vi "timeDvsfreqD_demo.vi"() -> ()   [LabVIEW 2009]
uses:
  <vilib>/imath/engines/lvmath2/RunTimeEngine/ErrorHandling/NIMS_Finalize Error.vi
  <vilib>/imath/engines/lvmath2/RunTimeEngine/Parser/MC_Version.vi
  <vilib>/imath/engines/lvmath2/RunTimeEngine/NodeEndStatement/NIMS_NodeEndStatement_Output.vi
  <instcachedir>/0/NIMS_NodeEndStatement_Output_53EC0D466D134D7ABD903AC30B43404B.lvgen/NIMS_NodeEndStatement_Output_53EC0D466D134D7ABD903AC30B43404B_001.vi
  <vilib>/imath/engines/lvmath/Functions/Error Handling/MergeErrorsWrapper.vi
  <vilib>/imath/engines/lvmath2/RunTimeEngine/NodeEndStatement/NIMS_NodeEndStatement_Get Vector.vi
  <instcachedir>/0/NIMS_NodeEndStatement_Get Vector_708AE642CFEE4B9892E482CBBBA3A4D6.lvgen/NIMS_NodeEndStatement_Get Vector_708AE642CFEE4B9892E482CBBBA3A4D6_000.vi
  <instcachedir>/0/NIMS_NodeEndStatement_Get Vector_708AE642CFEE4B9892E482CBBBA3A4D6.lvgen/NIMS_NodeEndStatement_Get Vector_708AE642CFEE4B9892E482CBBBA3A4D6_001.vi
  <vilib>/imath/engines/lvmath2/RunTimeEngine/RangeToken/NIMS_Range.vi
  <instcachedir>/0/NIMS_Range_08574DECC23E450FAF0AC0BC39E6BEA7.lvgen/NIMS_Range_08574DECC23E450FAF0AC0BC39E6BEA7_001.vi
  <vilib>/imath/engines/lvmath/Plug In/_Char/NIMS_CH_character datatype.ctl
  <vilib>/imathl/engines/lvmath/Functions/Error Handling/Create Error.vi
  <vilib>/imath/engines/lvmath2/RunTimeEngine/BuiltInFunctions/random/NIMS_random.vi
  <vilib>/imath/engines/lvmath/Plug In/_Char/NIMS_CH_Character RV to String.vi
  <vilib>/imath/engines/lvmath/Functions/Error Handling/MC_Error Cluster From Error Code.vi
  <vilib>/imath/engines/lvmath2/RunTimeEngine/BuiltInFunctions/abs/NIMS_abs(signed).vi
  <instcachedir>/0/NIMS_abs(signed)_C4FCB8E6058B49B797C7C8D53CA5F6EC.lvgen/NIMS_abs(signed)_C4FCB8E6058B49B797C7C8D53CA5F6EC_000.vi
  <vilib>/imath/engines/lvmath2/RunTimeEngine/BuiltInFunctions/fft/NIMS_fft(GV).vi
  <instcachedir>/0/NIMS_fft(GV)_4C6467FC22F84E4BA42517A07EF978B0.lvgen/NIMS_fft(GV)_4C6467FC22F84E4BA42517A07EF978B0_001.vi
  <vilib>/imath/engines/lvmath2/RunTimeEngine/ArithmeticOperatorToken/NIMS_ArithmeticOperator_plus.vi
  <instcachedir>/0/NIMS_ArithmeticOperator_plus_48B9519178ED42D7840F01273E784BFE.lvgen/NIMS_ArithmeticOperator_plus_48B9519178ED42D7840F01273E784BFE_008.vi
  <instcachedir>/0/NIMS_abs(signed)_C4FCB8E6058B49B797C7C8D53CA5F6EC.lvgen/NIMS_abs(signed)_C4FCB8E6058B49B797C7C8D53CA5F6EC_002.vi
  <vilib>/imath/engines/lvmath2/RunTimeEngine/BuiltInFunctions/fft/NIMS_fft(GM).vi
  <instcachedir>/0/NIMS_fft(GM)_D61006EB97DF48D4B7BC0A22887DF931.lvgen/NIMS_fft(GM)_D61006EB97DF48D4B7BC0A22887DF931_000.vi
panel:
  in  "nmag":dbl=1e-06 caption="Order of \nMagnitude \nof the \nNoise" format="%#_6p"
  in  "M1":dbl=10.0
  in  "N1":dbl=256.0
  out "Both Signals (Frequency Domain)":cluster{dbl[], dbl[]}[](graph)
  out "Both Signals (Time Domain)":cluster{dbl[], dbl[]}[](graph)
  out "Total Signal (Frequency Domain)":dbl[](graph)
  out "Total Signal (Time Domain)":dbl[](graph)
  out "Desired Signal (Frequency Domain)":dbl[](graph)
  out "Desired Signal (Time Domain)":dbl[](graph)
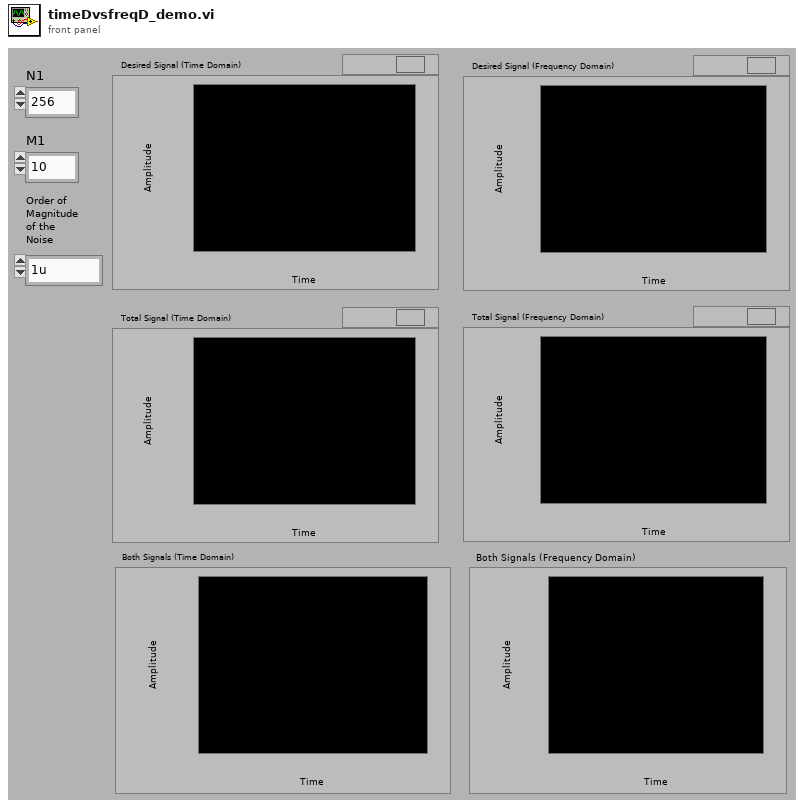
[diagram p1: front panel]
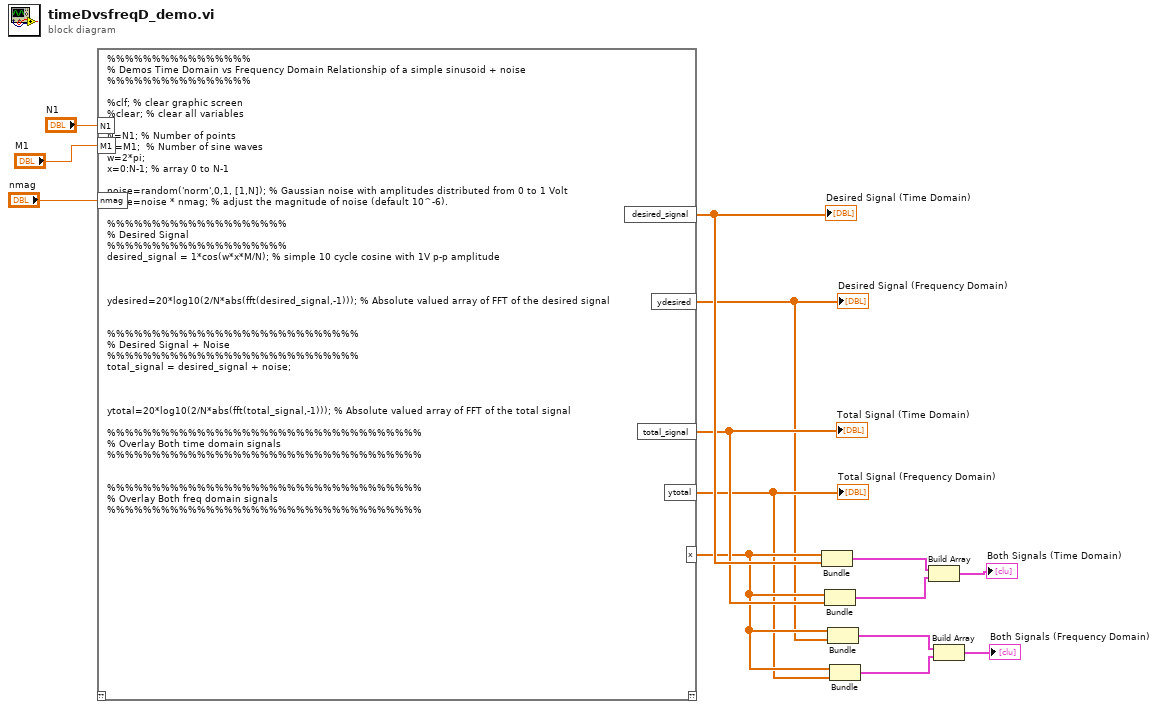
[diagram p0: block diagram]
diagram:
  n1 = mathscript code="%%%%%%%%%%%%%%%%\n% Demos Time Domain vs Frequency Domain Relationship of a simple sinusoid + noise\n%%%%%%%%%%%%%%%%\n\n%clf; % clear graphic screen\n%clear; % clear all variables\n\nN=N1; % Number of points\nM=M1;  % Number of sine waves\nw=2*pi; \nx=0:N-1; % array 0 to N-1\n\nnoise=random('norm',0,1, [1,N]); % Gaussian noise with amplitudes distributed from 0 to 1 Volt\nnoise=noise * nmag; % adjust the magnitude of noise (default 10^-6).\n\n%%%%%%%%%%%%%%%%%%%%\n% Desired Signal\n%%%%%%%%%%%%%%%%%%%%\ndesired_signal = 1*cos(w*x*M/N); % simple 10 cycle cosine with 1V p-p amplitude\n\n\n\nydesired=20*log10(2/N*abs(fft(desired_signal,-1))); % Absolute valued array of FFT of the desired signal \n\n\n%%%%%%%%%%%%%%%%%%%%%%%%%%%%\n% Desired Signal + Noise\n%%%%%%%%%%%%%%%%%%%%%%%%%%%%\ntotal_signal = desired_signal + noise;\n\n\n\nytotal=20*log10(2/N*abs(fft(total_signal,-1))); % Absolute valued array of FFT of the total signal \n\n%%%%%%%%%%%%%%%%%%%%%%%%%%%%%%%%%%%\n% Overlay Both time domain signals\n%%%%%%%%%%%%%%%%%%%%%%%%%%%%%%%%%%%\n\n\n%%%%%%%%%%%%%%%%%%%%%%%%%%%%%%%%%%%\n% Overlay Both freq domain signals\n%%%%%%%%%%%%%%%%%%%%%%%%%%%%%%%%%%%"("N1"="N1", "M1"="M1", "nmag"="nmag") -> ("desired_signal"=w14:dbl[], "ydesired"=w7:dbl[], "total_signal"=w13:dbl[], "ytotal"=w8:dbl[], "x"=w9:dbl[])  [unwired: 1 in, 1 out]
  "Desired Signal (Time Domain)" <- w14
  "Desired Signal (Frequency Domain)" <- w7
  "Total Signal (Time Domain)" <- w13
  "Total Signal (Frequency Domain)" <- w8
  n2 = Bundle(w9, w14) -> (w12:cluster{dbl[], dbl[]})  [unwired: 1 in]
  n3 = Bundle(w9, w13) -> (w11:cluster{dbl[], dbl[]})  [unwired: 1 in]
  n4 = Bundle(w9, w7) -> (w6:cluster{dbl[], dbl[]})  [unwired: 1 in]
  n5 = Bundle(w9, w8) -> (w5:cluster{dbl[], dbl[]})  [unwired: 1 in]
  n6 = Build Array(w12, w11) -> (→"Both Signals (Time Domain)":cluster{dbl[], dbl[]}[])
  n7 = Build Array(w6, w5) -> (→"Both Signals (Frequency Domain)":cluster{dbl[], dbl[]}[])
